vi "Dispose Server.vi"(8 "error in (no error)":errorcluster, 11 "Socket Server in":refnum<data-value>) -> (0 "error out":errorcluster)   [LabVIEW 2019, in "Socket API.lvlib" / "Socket Server.lvclass"]
uses:
  Socket Server.lvclass
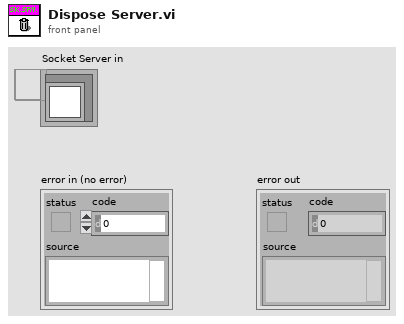
[diagram p1: front panel]
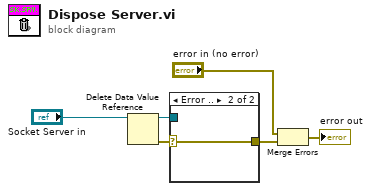
[diagram p0: block diagram]
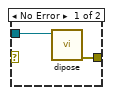
[diagram p2: hidden frame]
diagram:
  n1 = Delete Data Value Reference(data value reference="Socket Server in") -> (data value=w3:refnum<class "Socket Server.lvclass">, error out=w2:errorcluster)  [unwired: 1 in]
  n2 = case shown="Error .." w2 {
    selector: w2 -> [_ w9]
    tunnel: w3 -> [w8 _]
    tunnel: [w7 w9] -> w4
    frame No Error {
      n3 = call-dynamic "dipose.vi"("Socket Server in"=w8) -> ("error out"=w7:errorcluster)  [unwired: 10 in]
    }
    frame Error {
    }
  }
  n4 = Merge Errors("error in (no error)", w4) -> (→"error out":errorcluster)
